vi "Ctor.vi"(8 "error in (no error)":errorcluster) -> (0 "error out":errorcluster, 3 "Symbol Map out":refnum<class "Symbol Map.lvclass">)   [LabVIEW 2020, in "PicoG-ParserLexer.lvlib" / "Symbol Map.lvclass"]
uses:
  Symbol Map.lvclass
  Node/Node.lvclass
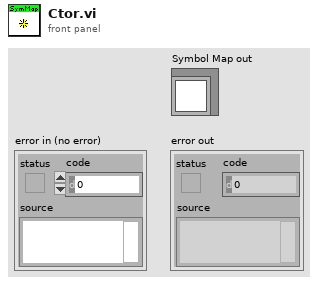
[diagram p1: front panel]
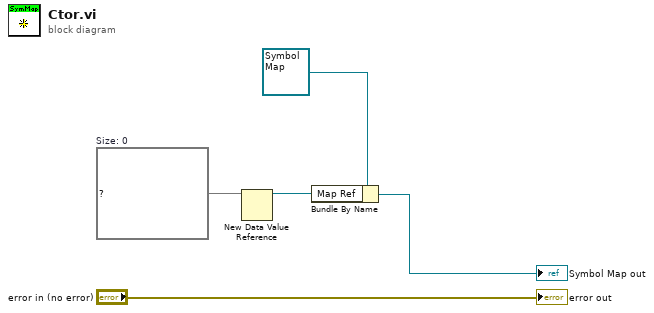
[diagram p0: block diagram]
diagram:
  w3 = map{string, refnum<data-value>} {}  # Size: 0
  n1 = New Data Value Reference(data value=w3) -> (data value reference=w1:refnum<data-value>)  [unwired: 1 in, 1 out]
  n2 = Bundle By Name(cluster=refnum<class "Symbol Map.lvclass"> refnum ("Symbol Map in"), "Map Ref"=w1) -> (→"Symbol Map out":refnum<class "Symbol Map.lvclass">)
  "error out" <- "error in (no error)"
